vi "Main.Reset DTC Enable Values.vi"(8 "error in":errorcluster, 11 "SimDTCs":T1[](array[typedef]) {"Data"."DM1 Ref"."Data Reference" format="%.0x"; "Data"."DM1 Enable Ref"."Data Reference" format="%.0x"; "Data"."DM2 Ref"."Data Reference" format="%.0x"; "Data"."DM2 Enable Ref"."Data Reference" format="%.0x"}) -> (0 "error out":errorcluster, 3 "SimDTCs":T1[](array[typedef]) {"Data"."DM1 Ref"."Data Reference" format="%.0x"; "Data"."DM1 Enable Ref"."Data Reference" format="%.0x"; "Data"."DM2 Ref"."Data Reference" format="%.0x"; "Data"."DM2 Enable Ref"."Data Reference" format="%.0x"})   [LabVIEW 2015, in "J1939 Addon Engine.lvlib"]
uses:
  J1939 Addon Engine.lvlib
  Types/Engine.DTC Settings.ctl
  Shared/Types/Compiled Simulated Settings.ctl
  <vilib>/NI Veristand/Custom Device API/Block Data Reference.ctl
  <vilib>/NI Veristand/Custom Device API/Data Reference.ctl
  Types/Engine.DTC FIFOs.ctl
  <vilib>/NI Veristand/Custom Device API/Global Data Refs.vi
  <vilib>/NI VeriStand/Custom Device API/Custom Device API.lvlib
  Shared/J1939 Addon Shared.lvlib
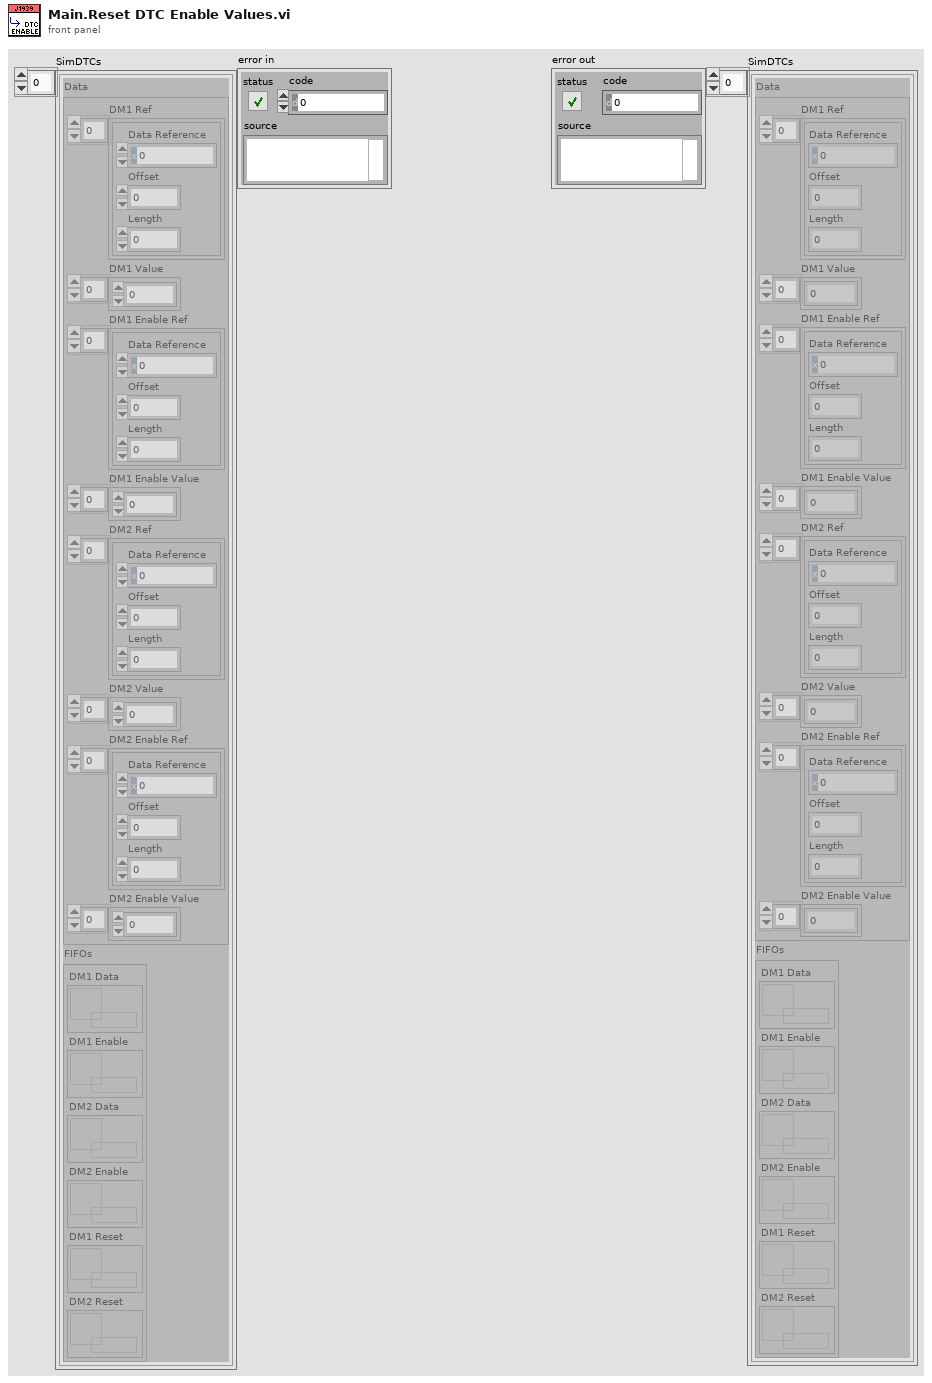
[diagram p1: front panel]
types:
  T1 = typedef "J1939 Addon Engine.lvlib/Engine.DTC Settings.ctl" = cluster{"Data":T2, "FIFOs":T5}
  T2 = typedef "J1939 Addon Shared.lvlib/Compiled Simulated Settings.ctl" = cluster{"DM1 Ref":T3[], "DM1 Value":dbl[], "DM1 Enable Ref":T3[], "DM1 Enable Value":dbl[], "DM2 Ref":T3[], "DM2 Value":dbl[], "DM2 Enable Ref":T3[], "DM2 Enable Value":dbl[]}
  T3 = typedef "Custom Device API.lvlib/Block Data Reference.ctl" = cluster{"Data Reference":T4, "Offset":u64, "Length":u64}
  T4 = typedef "Custom Device API.lvlib/Data Reference.ctl" = i32
  T5 = typedef "J1939 Addon Engine.lvlib/Engine.DTC FIFOs.ctl" = cluster{"DM1 Data":refnum<k33>, "DM1 Enable":refnum<k33>, "DM2 Data":refnum<k33>, "DM2 Enable":refnum<k33>, "DM1 Reset":refnum<k33>, "DM2 Reset":refnum<k33>}
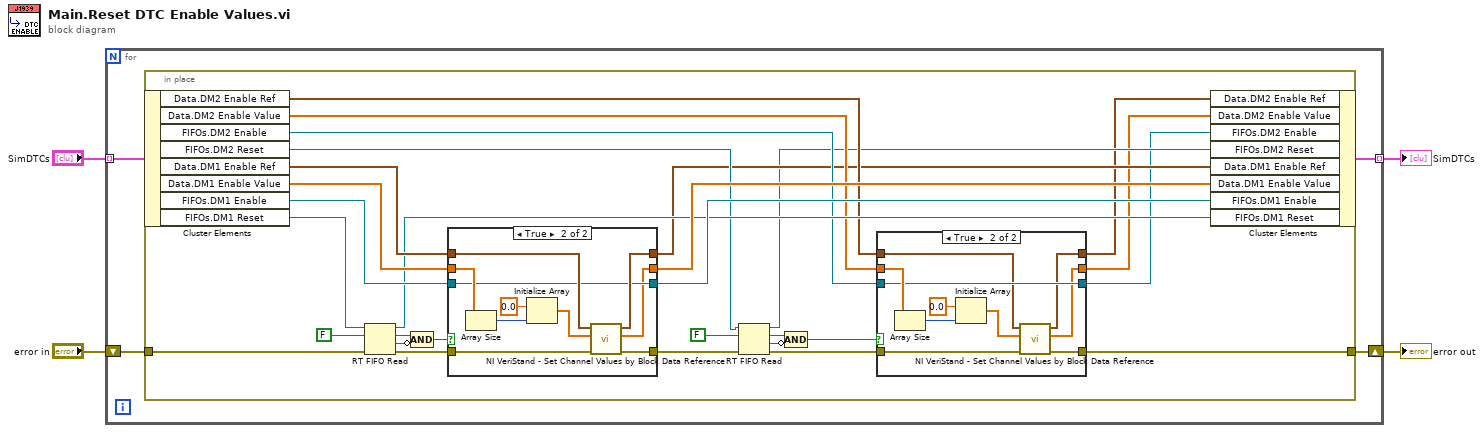
[diagram p0: block diagram]
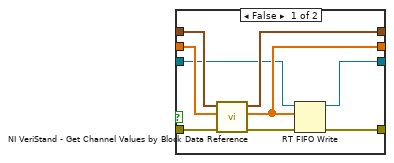
[diagram p2: hidden frame]
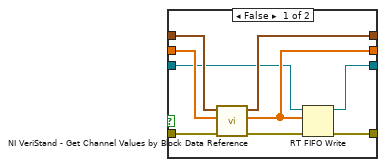
[diagram p3: hidden frame]
diagram:
  n1 = for {
    tunnel: "SimDTCs" -> [w8] mode=indexing
    shift-right: [w7] -> w2
    shift-left: "error in" -> [w5]
    tunnel: [w6] -> w1 mode=indexing
    n2 = in-place {
      in-place-border: [w10] -> w7
      in-place-border: w5 -> [w9]
      n3 = in-place-cluster #1(w8) -> ("Data.DM2 Enable Ref"=w16:T3[], "Data.DM2 Enable Value"=w17:dbl[], "FIFOs.DM2 Enable"=w18:refnum<k33>, "FIFOs.DM2 Reset"=w19:refnum<k33>, "Data.DM1 Enable Ref"=w32:T3[], "Data.DM1 Enable Value"=w31:dbl[], "FIFOs.DM1 Enable"=w29:refnum<k33>, "FIFOs.DM1 Reset"=w37:refnum<k33>)
      n4 = RT FIFO Read(0:w37, 1:FALSE ("element"), 3:w9) -> (8:w20:refnum<k33>, 9:w36:bool, 10:w35:bool, 11:w30:errorcluster)  [unwired: 1 in, 1 out]
      n5 = Compound Arithmetic op=AND(w36, invert w35) -> (w33:bool)
      n6 = case shown="True" w33 {
        tunnel: w32 -> [w65 w70]
        tunnel: w31 -> [w64 w75]
        tunnel: w30 -> [w63 w72]
        tunnel: w29 -> [w58 w68]
        tunnel: [w61 w66] -> w28
        tunnel: [w60 w71] -> w23
        tunnel: [w57 w68] -> w27
        tunnel: [w59 w69] -> w15
        frame False {
          n7 = call <vilib>:"NI VeriStand - Get Channel Values by Block Data Reference.vi"("error in (no error)"=w63, "Values Array in"=w64, "Block Data Ref"=w65) -> ("error out"=w62:errorcluster, "Values Array out"=w61:dbl[], "Block Data Ref dup"=w59:T3[])  [unwired: 6 in]
          n8 = RT FIFO Write(0:w58, 1:w61, 3:w62) -> (8:w57:refnum<k33>, 11:w60:errorcluster)  [unwired: 2 in, 2 out]
        }
        frame True {
          n9 = Array Size(array=w75) -> (size(s)=w74:i32)
          n10 = Initialize Array(0.0 ("element"), w74) -> (w67:dbl[])
          n11 = call <vilib>:"NI VeriStand - Set Channel Values by Block Data Reference.vi"("error in (no error)"=w72, "Values Array in"=w67, "Block Data Ref"=w70) -> ("error out"=w71:errorcluster, "Values Array out"=w66:dbl[], "Block Data Ref dup"=w69:T3[])  [unwired: 6 in]
        }
      }
      n12 = RT FIFO Read(0:w19, 1:FALSE ("element"), 3:w23) -> (8:w14:refnum<k33>, 9:w24:bool, 10:w25:bool, 11:w22:errorcluster)  [unwired: 1 in, 1 out]
      n13 = Compound Arithmetic op=AND(w24, invert w25) -> (w21:bool)
      n14 = case shown="True" w21 {
        tunnel: w16 -> [w46 w50]
        tunnel: w17 -> [w45 w56]
        tunnel: w22 -> [w44 w52]
        tunnel: w18 -> [w39 w53]
        tunnel: [w42 w47] -> w12
        tunnel: [w41 w51] -> w10
        tunnel: [w38 w53] -> w11
        tunnel: [w40 w49] -> w13
        frame False {
          n15 = call <vilib>:"NI VeriStand - Get Channel Values by Block Data Reference.vi"("error in (no error)"=w44, "Values Array in"=w45, "Block Data Ref"=w46) -> ("error out"=w43:errorcluster, "Values Array out"=w42:dbl[], "Block Data Ref dup"=w40:T3[])  [unwired: 6 in]
          n16 = RT FIFO Write(0:w39, 1:w42, 3:w43) -> (8:w38:refnum<k33>, 11:w41:errorcluster)  [unwired: 2 in, 2 out]
        }
        frame True {
          n17 = Array Size(array=w56) -> (size(s)=w55:i32)
          n18 = Initialize Array(0.0 ("element"), w55) -> (w48:dbl[])
          n19 = call <vilib>:"NI VeriStand - Set Channel Values by Block Data Reference.vi"("error in (no error)"=w52, "Values Array in"=w48, "Block Data Ref"=w50) -> ("error out"=w51:errorcluster, "Values Array out"=w47:dbl[], "Block Data Ref dup"=w49:T3[])  [unwired: 6 in]
        }
      }
      n20 = in-place-cluster #1("Data.DM2 Enable Ref"=w13, "Data.DM2 Enable Value"=w12, "FIFOs.DM2 Enable"=w11, "FIFOs.DM2 Reset"=w14, "Data.DM1 Enable Ref"=w15, "Data.DM1 Enable Value"=w28, "FIFOs.DM1 Enable"=w27, "FIFOs.DM1 Reset"=w20) -> (w6:T1)
    }
  }
  "error out" <- w2
  "SimDTCs" <- w1
